vi "ActionVIOnCompile.vi"(8 "error in":errorcluster, 11 "Device Item Ref in":u64 format="%.0x") -> (0 "error out":errorcluster)   [LabVIEW 2026, in "SystemMonitor Configuration.lvlib"]
uses:
  SystemMonitor Configuration.lvlib
  <vilib>/NI VeriStand/Custom Device API/Custom Device API.lvlib
  NationalInstruments.VeriStand.SystemDefinitionAPI
  <vilib>/NI VeriStand/Custom Device API/Set Item Property (Variant).vi
  <userlib>/Custom Device Interfaces_v1.lvlibp/CustomDeviceDeploymentHooks/Custom Device Deployment Hooks.lvclass
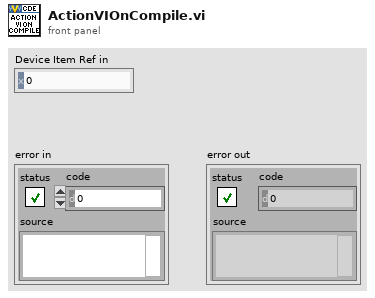
[diagram p1: front panel]
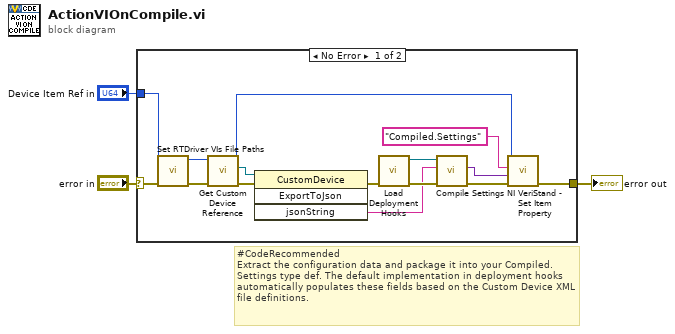
[diagram p0: block diagram]
diagram:
  # "#CodeRecommended\nExtract the configuration data and package it into your Compiled.Settings type def. The default implementation in deployment hooks automatically populates these fields based on the Custom Device XML file definitions."
  n1 = case shown="No Error" "error in" {
    selector: "error in" -> [w18 w19]
    tunnel: [w10 w19] -> w2
    tunnel: "Device Item Ref in" -> [w17 _]
    frame No Error {
      n2 = call "Set RTDriver VIs File Paths.vi"("error in"=w18, "Item Ref in"=w17) -> ("error out"=w4:errorcluster, "Item Ref out"=w5:u64)  [unwired: 8 in]
      n3 = call "Get Custom Device Reference.vi"("error in"=w4, "Item Ref in"=w5) -> ("error out"=w6:errorcluster, "Custom Device"=w7:refnum<k24>, "Item Ref out"=w8:u64)  [unwired: 7 in]
      n4 = invoke class="CustomDevice" method="ExportToJson"(reference=w7, error in=w6) -> (error out=w11:errorcluster, "jsonString"=w9:string)  [unwired: 2 in, 2 out]
      n5 = call "Load Deployment Hooks.vi"("error in"=w11) -> ("error out"=w16:errorcluster, "Custom Device Deployment Hooks out"=w13:refnum<class "Custom Device Deployment Hooks.lvclass">)  [unwired: 9 in]
      n6 = call-dynamic "Compile Settings.vi"("error in"=w16, "Settings(JSON)"=w9, "Custom Device Deployment Hooks in"=w13) -> ("error out"=w15:errorcluster, "Compiled Settings"=w12:variant)  [unwired: 6 in, 1 out]
      n7 = call-poly <vilib>:"NI VeriStand - Set Item Property.vi"("error in (no error)"=w15, "Value"=w12, "Property Name"="Compiled.Settings" ("Compiled.Settings"), "Item Ref in"=w8) -> ("error out"=w10:errorcluster)  [unwired: 5 in, 2 out]
    }
    frame Error {
    }
  }
  "error out" <- w2
